vi "uService Class Finder.vi"(8 "error in (no error)":errorcluster, 9 "uService ID in":string, 10 "uService Class name":string, 11 "Guardian in":refnum<class "Guardian.lvclass">) -> (0 "error out":errorcluster, 1 "uService ID out":string, 2 "uService out":refnum<class "Father of all uServices.lvclass">, 3 "Guardian out":refnum<class "Guardian.lvclass">)   [LabVIEW 2026, in "TALOS.lvlib" / "Guardian.lvlib" / "Guardian.lvclass"]
doc: "This VI loks in the current application folder for a uService with the corresponding name, and return the appropriate class object. It also checks if the class found is a children of uService Father and if the ID is already in the system, and add a number to make it unique."
uses:
  Guardian.lvclass
  Father of all uServices/Father of all uServices/Father of all uServices.lvclass
  Classes/uService List/uService List.lvclass/uService List.ctl
  Ancestor/Ancestor/Ancestor.lvclass/Ancestor.ctl
  Classes/uService List/Get all IDs.vi
  FGV/Error Memory/Get Error Description.vi
  Support VIs/Get PC name.vi
  Ancestor/Ancestor/Read ID.vi
  Support VIs/Get Class Name.vi
  <vilib>/Utility/error.llb/Clear Errors.vi
  FGV/Error Memory/Error Memory Core.vi
  <vilib>/AdvancedString/Delimited String to 1D String Array.vi
  <vilib>/AdvancedString/Delimited String to 1D String Array (string).vi
  FGV/Error Memory/Error Crt Lvl checker.vi
  FGV/Error Memory/Error Memory Core.vi/40c8088d-b597-4017-91af-faa98e00292e.vi
  FGV/Error Memory/Error Memory Core.vi/d4a3ab98-063c-4e44-b43d-fbdcfe6c2be2.vi
  Support VIs/Global Memory.vi
  <vilib>/Utility/LVClass/Get LV Class Name.vi
  Support VIs/Read CSV worksheet.vi
  Support VIs/Global Constants.vi
  <vilib>/Utility/error.llb/General Error Handler.vi
  Support VIs/Error Log.vi
  Ancestor/Ancestor/Ancestor.lvclass
  <vilib>/Comparison/Equal/Equal Functor/Equal Functor.lvclass
  Classes/uService List/uService List.lvclass
  TALOS.lvlib
  <vilib>/Utility/LVLibp/NI_PackedLibraryUtility.lvlib
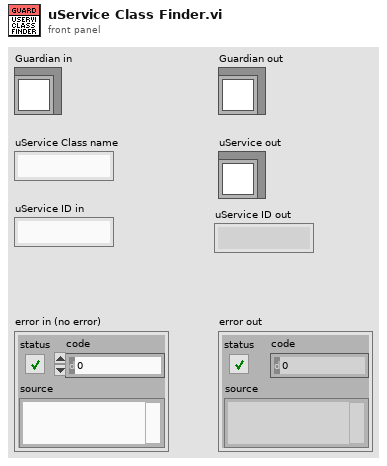
[diagram p1: front panel]
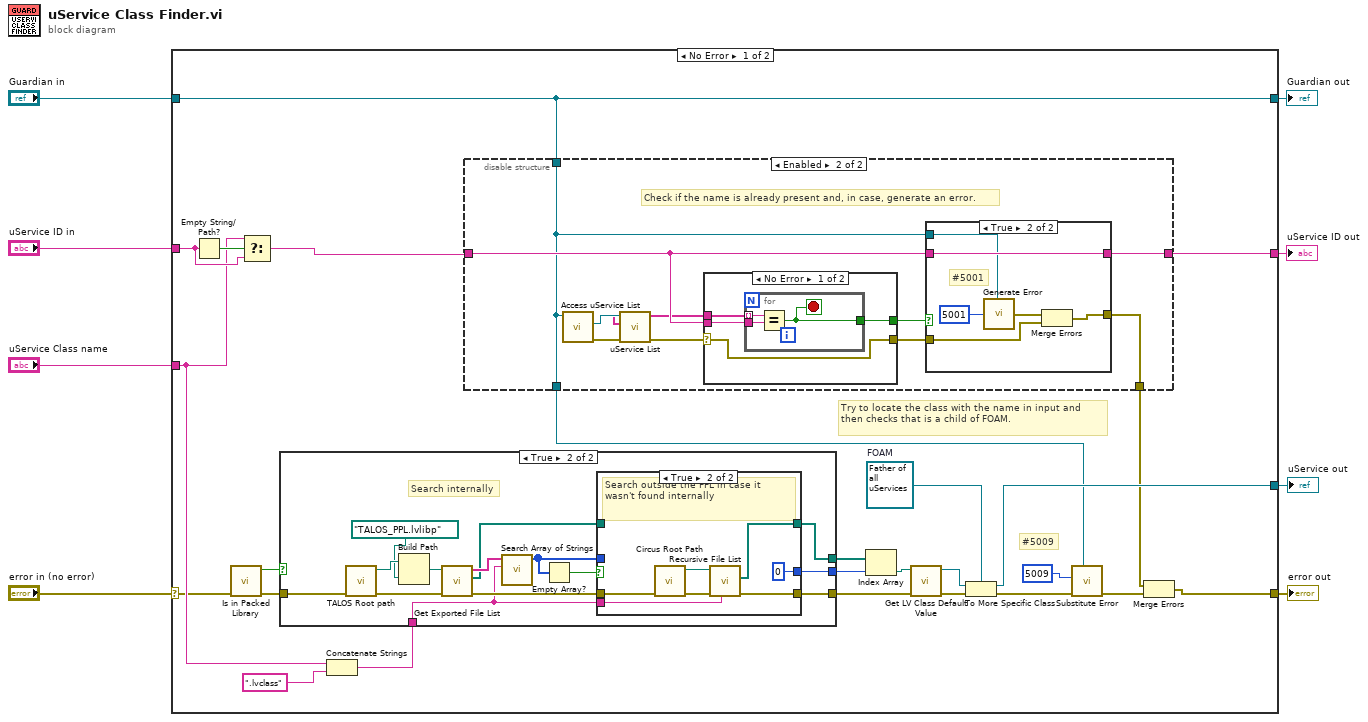
[diagram p0: block diagram]
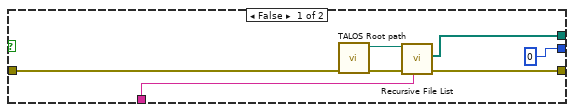
[diagram p2: hidden frame]
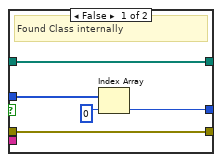
[diagram p3: hidden frame]
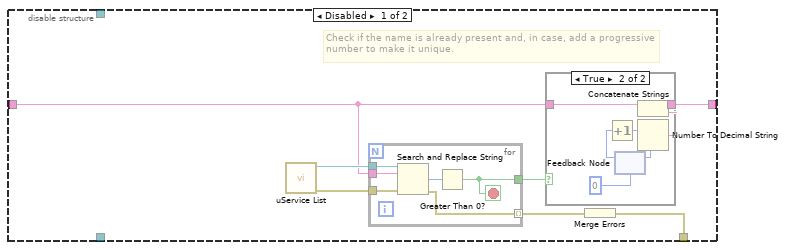
[diagram p4: hidden frame]
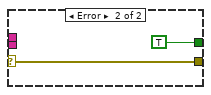
[diagram p6: hidden frame]
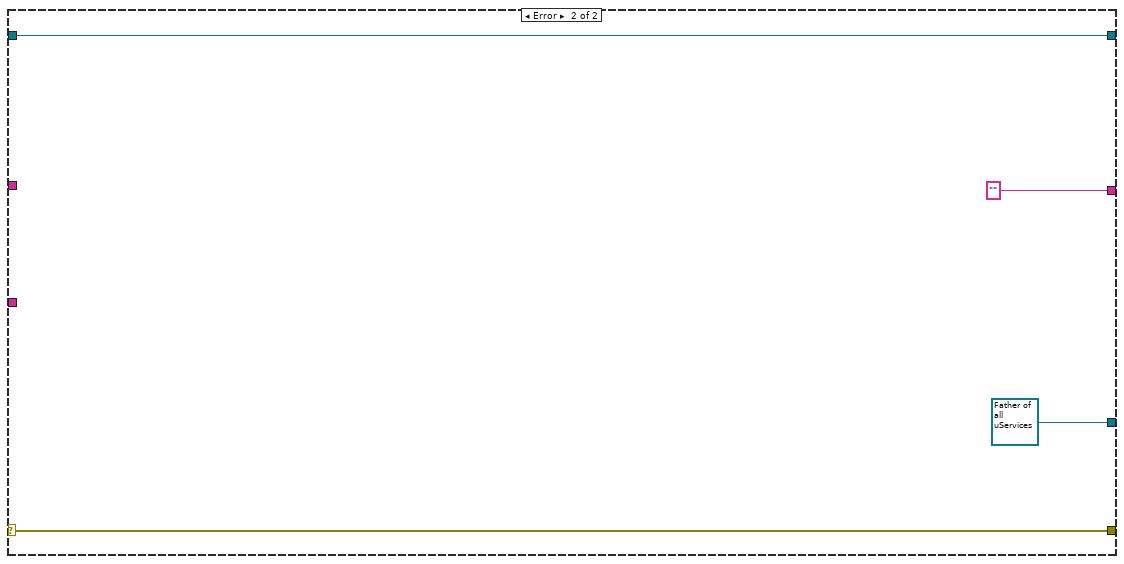
[diagram p8: hidden frame]
diagram:
  n1 = case shown="No Error" "error in (no error)" {
    selector: "error in (no error)" -> [w11 w117]
    tunnel: [w29 refnum<class "Father of all uServices.lvclass"> refnum ("uService Template")] -> w7
    tunnel: "uService Class name" -> [w22 _]
    tunnel: [w27 "" ("uService Class name")] -> w5
    tunnel: [w26 w117] -> w4
    tunnel: "uService ID in" -> [w23 _]
    tunnel: "Guardian in" -> [w13 w114]
    tunnel: [w13 w114] -> w1
    frame No Error {
      w30 = refnum<class "Father of all uServices.lvclass"> refnum  # FOAM
      # "#5009"
      # "Try to locate the class with the name in input and then checks that is a child of FOAM."
      n2 = Empty String/Path?(string/path=w23) -> (empty?=w24:bool)
      n3 = call "Is in Packed Library.vi"("error in (no error)"=w11) -> ("error out"=w10:errorcluster, "Is In Packed Library"=w9:bool)  [unwired: 9 in]
      n4 = Select(t=w22, s=w24, f=w23) -> (s? t:f=w21:string)
      n5 = Concatenate Strings(w22, ".lvclass" ("pattern")) -> (w20:string)
      n6 = case shown="True" w9 {
        tunnel: w10 -> [w40 w49]
        tunnel: w20 -> [w39 w43]
        tunnel: [w36 w44] -> w19
        tunnel: [w35 w47] -> w18
        tunnel: [0 ("index") w45] -> w17
        frame False {
          n7 = call "TALOS Root path.vi"("error in (no error)"=w40) -> ("error out"=w38:errorcluster, "TALOS Root Path"=w37:path)  [unwired: 9 in]
          n8 = call <vilib>:"Recursive File List.vi"("pattern"=w39, "error in (no error)"=w38, "Folder Path"=w37) -> ("error out"=w36:errorcluster, "All Files in Dir"=w35:path[])  [unwired: 4 in, 3 out]
        }
        frame True {
          # "Search internally"
          n9 = call "TALOS Root path.vi"("error in (no error)"=w49) -> ("error out"=w52:errorcluster, "TALOS Root Path"=w54:path)  [unwired: 9 in]
          n10 = Build Path(base path=w54, name or relative path=path "TALOS_PPL.lvlibp") -> (appended path=w53:path)
          n11 = call <vilib>:"Get Exported File List.vi"("error in (no error)"=w52, "packed library path"=w53) -> ("error out"=w48:errorcluster, "paths"=w46:path[], "qualified names"=w51:string[])  [unwired: 7 in]
          n12 = call "Search Array of Strings.vi"("search string"=w43, "Search array"=w51) -> ("indices"=w42:i32[])  [unwired: 8 in, 1 out]
          n13 = Empty Array?(array=w42) -> (empty?=w41:bool)
          n14 = case shown="True" w41 {
            tunnel: w46 -> [w59 _]
            tunnel: [w59 w62] -> w47
            tunnel: [w55 0] -> w45
            tunnel: [w58 w61] -> w44
            tunnel: w43 -> [_ w63]
            tunnel: w42 -> [w57 _]
            tunnel: w48 -> [w58 w64]
            frame False {
              # "Found Class internally"
              n15 = Index Array(array=w57, index=0) -> (element=w55:i32)
            }
            frame True {
              # "Search outside the PPL in case it wasn't found internally"
              n16 = call "Circus Root Path.vi"("error in (no error)"=w64) -> ("error out"=w66:errorcluster, "Circus Root Path"=w65:path)  [unwired: 9 in]
              n17 = call <vilib>:"Recursive File List.vi"("pattern"=w63, "error in (no error)"=w66, "Folder Path"=w65) -> ("error out"=w61:errorcluster, "All Files in Dir"=w62:path[])  [unwired: 4 in, 3 out]
            }
          }
        }
      }
      n18 = disable-structure "Diagram Disable Structure" shown="Enabled" {
        disable-tunnel: w21 -> [w71 w96]
        disable-tunnel: [w70 w95] -> w27
        disable-tunnel: [w67 w93] -> w25
        disable-tunnel: w13 -> [_ w89]
        disable-tunnel: [_ w89] -> w12
        frame Disabled {
          # "Check if the name is already present and, in case, add a progressive number to make it unique."
          n19 = call-poly "uService List.vi"() -> ("error out"=w69:errorcluster, "uService List out"=w73:refnum<class "uService List.lvclass">)  [unwired: 9 in, 1 out]
          n20 = for {
            tunnel: w73 -> [w86]
            tunnel: w71 -> [w85]
            tunnel: [w83] -> w72
            tunnel: w69 -> [w82]
            tunnel: [w81] -> w68 mode=indexing
            stop <- w83 stop-if-true
            n21 = Search and Replace String(input string=w86, search string=w85, error in=w82) -> (number of replacements=w84:i32, error out=w81:errorcluster)  [unwired: 5 in, 2 out]
            n22 = Greater Than 0?(x=w84) -> (x > 0?=w83:bool)
          }
          n23 = case shown="True" w72 {
            tunnel: w71 -> [w74 w78]
            tunnel: [w74 w77] -> w70
            frame False {
            }
            frame True {
              n24 = feedback #1(0) -> (w75:i32)
              n25 = Increment(x=w75) -> (x+1=w76:i32)
              n26 = feedback-in #1(w76) -> ()
              n27 = Number To Decimal String(number=w76) -> (decimal integer string=w79:string)  [unwired: 1 in]
              n28 = Concatenate Strings(w78, w79) -> (w77:string)
            }
          }
          n29 = Merge Errors(w68) -> (w67:errorcluster)
        }
        frame Enabled {
          # "Check if the name is already present and, in case, generate an error."
          n30 = call-dynamic "Access uService List.vi"("Ancestor in"=w89) -> ("error out"=w92:errorcluster, "uService List out"=w91:refnum<class "uService List.lvclass">)  [unwired: 8 in, 1 out]
          n31 = call-poly "uService List.vi"("error in (no error)"=w92, "uService List"=w91) -> ("error out"=w94:errorcluster, "All IDs"=w90:string[])  [unwired: 7 in, 1 out]
          n32 = case shown="No Error" w94 {
            selector: w94 -> [w97 w105]
            tunnel: w96 -> [w100 _]
            tunnel: w90 -> [w99 _]
            tunnel: [w98 TRUE] -> w88
            tunnel: [w97 w105] -> w87
            frame No Error {
              n33 = for {
                tunnel: w99 -> [w103] mode=indexing
                tunnel: w100 -> [w102]
                tunnel: [w101] -> w98
                stop <- w101 stop-if-true
                n34 = Equal?(x=w103, y=w102) -> (x = y?=w101:bool)
              }
            }
            frame Error {
            }
          }
          n35 = case shown="True" w88 {
            tunnel: w96 -> [w107 w113]
            tunnel: [w107 w113] -> w95
            tunnel: [w106 w109] -> w93
            tunnel: w89 -> [_ w111]
            tunnel: w87 -> [w106 w108]
            frame False {
            }
            frame True {
              # "#5001"
              n36 = call "Generate Error.vi"("Class"=w111, "Error Code"=5001) -> ("error out"=w110:errorcluster)  [unwired: 5 in]
              n37 = Merge Errors(w110, w108) -> (w109:errorcluster)
            }
          }
        }
      }
      n38 = Index Array(array=w18, index=w17) -> (element=w32:path)
      n39 = call <vilib>:"Get LV Class Default Value.vi"("error in (no error)"=w19, "class path"=w32) -> ("error out"=w31:errorcluster, "object"=w28:refnum<class>)  [unwired: 8 in]
      n40 = To More Specific Class(target class=w30, reference=w28, error in=w31) -> (specific class reference=w29:refnum<class "Father of all uServices.lvclass">, error out=w16:errorcluster)
      n41 = call "Substitute Error.vi"("LabVIEW Object"=w12, "error in (no error)"=w16, "Error Code"=5009) -> ("error out"=w14:errorcluster)  [unwired: 8 in]
      n42 = Merge Errors(w25, w14) -> (w26:errorcluster)
    }
    frame Error {
    }
  }
  "error out" <- w4
  "uService out" <- w7
  "uService ID out" <- w5
  "Guardian out" <- w1
